vi "Live img palette disabled.vi"(8 "error in (no error)":errorcluster, 11 "Left/Right":T1) -> (0 "error out":errorcluster)   [LabVIEW 2013]
uses:
  Typedefs/Left-Right enum.ctl
  Globals/gl_Windows Ctrl refs.vi
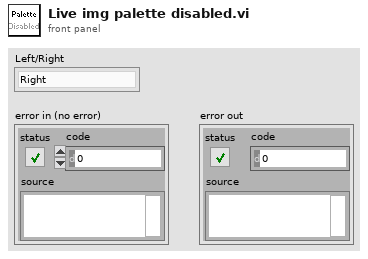
[diagram p1: front panel]
types:
  T1 = typedef "Left-Right enum.ctl" = enum16{"Right", "Left"}
  T2 = typedef "Live window-ctrl refs.ctl" = cluster{"This VI":refnum<vi>, "Pane":refnum<vi>, "Snapshot":refnum<vi>, "Left Image Palette":refnum<vi>, "Right Image Palette":refnum<vi>, "Left Channel":refnum<vi>, "Right Channel":refnum<vi>, "Left image intensity":refnum<vi>, "Right image intensity":refnum<vi>, "Left Image Display":T3, "Right Image Display":T3, "Refresh rate ind (Hz)":refnum<vi>, "Acq rate ind (Hz)":refnum<vi>, "Stop (ind)":refnum<vi>}
  T3 = typedef "Image display ref.ctl" = refnum<vi>
  T4 = typedef "Channel Selector.ctl" = enum16{"Red Channel", "Green Channel", "Blended"}
  T5 = enum8{"Enabled", "Disabled", "Disabled and Grayed Out"}
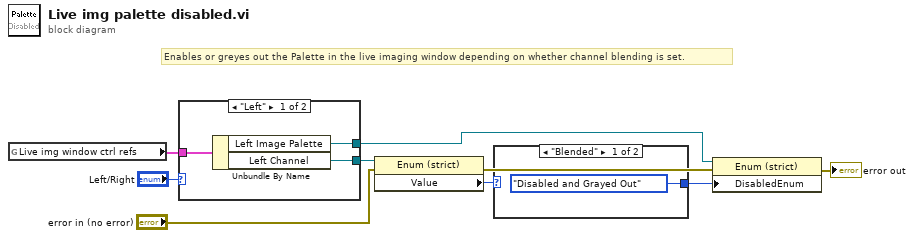
[diagram p0: block diagram]
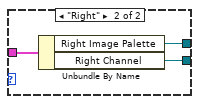
[diagram p2: hidden frame]
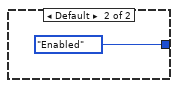
[diagram p3: hidden frame]
diagram:
  # "Enables or greyes out the Palette in the live imaging window depending on whether channel blending is set."
  n1 = global read "gl_Windows Ctrl refs.vi" "Live img window ctrl refs"() -> (w3:T2)
  n2 = case shown="\"Left\"" "Left/Right" {
    tunnel: [w12 w15] -> w6
    tunnel: w3 -> [w11 w14]
    tunnel: [w10 w13] -> w5
    frame "Left" {
      n3 = Unbundle By Name(w11) -> ("Left Image Palette"=w12:refnum<vi>, "Left Channel"=w10:refnum<vi>)
    }
    frame "Right" {
      n4 = Unbundle By Name(w14) -> ("Right Image Palette"=w15:refnum<vi>, "Right Channel"=w13:refnum<vi>)
    }
  }
  n5 = property on="Property Node" class="Enum (strict)"(reference=w5, error in="error in (no error)") -> (error out=w7:errorcluster, "Value"=w1:T4)  [unwired: 1 out]
  n6 = case shown="\"Blended\"" w1 {
    tunnel: [T5."Disabled and Grayed Out" ("Disabled") T5."Enabled" ("Disabled")] -> w2
    frame "Blended" {
    }
    frame Default {
    }
  }
  n7 = property on="Property Node" class="Enum (strict)"(reference=w6, error in=w7, "DisabledEnum"=w2) -> (error out=→"error out":errorcluster)  [unwired: 1 out]
